vi "PH_SystemInformation.ProcEvents.vi"(0 "i ref in":refnum<vi>, 5 "error in (no error)":errorcluster) -> (14 "i ref out":refnum<vi>, 19 "error out":errorcluster)   [LabVIEW 2014, in "PH_SystemInformation.lvlib"]
doc: "This method is used to define the events the object will listen to. Add your own events here."
uses:
  PH_SystemInformation.lvlib
  PH_Common/DIM/PH_DIM.Event Declarer.ctl
  CS_Core/BaseProcess/BaseProcess.lvlib
  PH_Common/PH_Common.lvlib
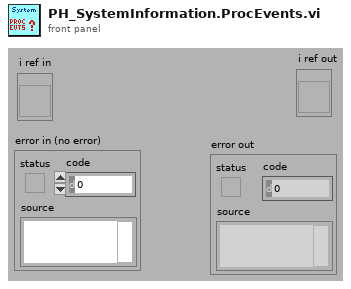
[diagram p1: front panel]
types:
  T1 = typedef "PH_Common.lvlib/PH_DIM.Event Declarer.ctl" = cluster{"Service Name":string, "Selector":string}
  T2 = typedef "PH_SystemInformation.lvlib/PH_SystemInformation.i attribute.ctl" = cluster{"Laser Enabling":cluster{"GUI Ref":refnum<vi>, "Enabling State":T3}, "PreAmp Enabling":cluster{"GUI Ref":refnum<vi>, "Enabling State":T3}, "MainAmp Enabling":cluster{"GUI Ref":refnum<vi>, "Enabling State":T3}, "Emergency Off":cluster{"GUI Ref":refnum<vi>, "State":enum16{"no info", "off/false", "Alarm"}}, "Enabling Exp. 1":cluster{"GUI Ref":refnum<vi>, "Enabling State":T3}, "Enabling Exp. 2":cluster{"GUI Ref":refnum<vi>, "Enabling State":T3}, "Enabling Exp. 3":cluster{"GUI Ref":refnum<vi>, "Enabling State":T3}, "Enabling Exp. 4":cluster{"GUI Ref":refnum<vi>, "Enabling State":T3}, "Timing Mode":cluster{"GUI Ref":refnum<vi>, "PHELIX_Timing_Mode":enum32{"10 Hz", "0.5 Hz", "Shot"}}}
  T3 = typedef "PH_SystemInformation.lvlib/PH_SystemInformationEnabling State.ctl" = i32
  T4 = typedef "BaseProcess.lvlib/BaseProcess.event definition.ctl" = cluster{"CAEEvtDef":T5, "Data Descriptor":T6}
  T5 = typedef "CAEObj.lvlib/CAEObj.event definition.ctl" = cluster{"URL":string, "enable":bool, "ignoreResID":bool}
  T6 = typedef "BaseProcess.lvlib/BaseProcess.descriptor string definition.ctl" = string
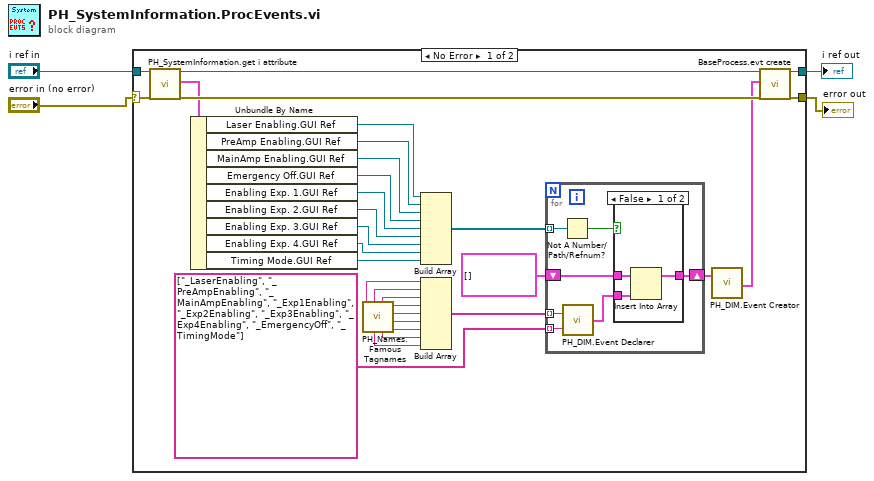
[diagram p0: block diagram]
diagram:
  n1 = case shown="No Error" "error in (no error)" {
    selector: "error in (no error)" -> [w28 w47]
    tunnel: "i ref in" -> [w35 w48]
    tunnel: [w32 w47] -> w3
    tunnel: [w31 w48] -> w2
    frame No Error {
      n2 = call "PH_SystemInformation.get i attribute.vi"("i ref in"=w35, "error in (no error)"=w28) -> ("i ref out"=w33:refnum<vi>, "i attribute"=w17:T2, "error out"=w34:errorcluster)  [unwired: 15 in]
      n3 = Unbundle By Name(w17) -> ("Laser Enabling.GUI Ref"=w26:refnum<vi>, "PreAmp Enabling.GUI Ref"=w25:refnum<vi>, "MainAmp Enabling.GUI Ref"=w24:refnum<vi>, "Emergency Off.GUI Ref"=w23:refnum<vi>, "Enabling Exp. 1.GUI Ref"=w22:refnum<vi>, "Enabling Exp. 2.GUI Ref"=w21:refnum<vi>, "Enabling Exp. 3.GUI Ref"=w20:refnum<vi>, "Enabling Exp. 4.GUI Ref"=w19:refnum<vi>, "Timing Mode.GUI Ref"=w18:refnum<vi>)
      n4 = call "PH_Names.Famous Tagnames.vi"() -> ("Laser Enabling.DIM Service Name"=w13:string, "PreAmp Enabling.DIM Service Name"=w12:string, "Timing Mode.DIM Service Name"=w5:string, "MainAmp Enabling.DIM Service Name"=w11:string, "Enabling Exp. 1.DIM Service Name"=w10:string, "Enabling Exp. 2.DIM Service Name"=w9:string, "Emergency Off.DIM Service Name"=w6:string, "Enabling Exp. 3.DIM Service Name"=w8:string, "Enabling Exp. 4.DIM Service Name"=w7:string)  [unwired: 2 in]
      n5 = Build Array(w26, w25, w24, w23, w22, w21, w20, w19, w18) -> (w14:refnum<vi>[])
      n6 = Build Array(w13, w12, w11, w10, w9, w8, w7, w6, w5) -> (w30:string[])
      n7 = for {
        tunnel: w30 -> [w41] mode=indexing
        tunnel: string[] ["_LaserEnabling", "_PreAmpEnabling", "_MainAmpEnabling", "_Exp1Enabling", "_Exp2Enabling", "_Exp3Enabling", "_Exp4Enabling", "_EmergencyOff", "_TimingMode"] -> [w40] mode=indexing
        shift-right: [w39] -> w16
        shift-left: T1[] [] -> [w38]
        tunnel: w14 -> [w37] mode=indexing
        n8 = Not A Number/Path/Refnum?(number/path/refnum=w37) -> (NaN/Path/Refnum?=w36:bool)
        n9 = call "PH_DIM.Event Declarer.vi"("Selector"=w40, "Service Name"=w41) -> ("declared DIM Event"=w42:T1)
        n10 = case shown="False" w36 {
          tunnel: w42 -> [w43 _]
          tunnel: [w45 w46] -> w39
          tunnel: w38 -> [w44 w46]
          frame False {
            n11 = Insert Into Array(array=w44, new element=w43) -> (w45:T1[])  [unwired: 1 in]
          }
          frame True {
          }
        }
      }
      n12 = call "PH_DIM.Event Creator.vi"("Trendmessage Services"=w16) -> ("DIM Service Events"=w27:T4[])  [unwired: 18 in]
      n13 = call "BaseProcess.evt create.vi"("i ref in"=w33, "newEvents"=w27, "error in (no error)"=w34) -> ("i ref out"=w31:refnum<vi>, "error out"=w32:errorcluster)  [unwired: 13 in, 2 out]
    }
    frame Error {
    }
  }
  "i ref out" <- w2
  "error out" <- w3
